vi "niFpgaDiscreteControlFilterTemplate.vi"(0 "input":fxp<+/-,16,16>, 1 "reset":bool) -> (4 "output":fxp<+/-,16,16>)   [LabVIEW 2017]
doc: "Applies a fifth-order low-pass integer FIR filter to the input data. The filter cut-off frequency is 1/10 of the sample frequency of the <B>input</B>. Use the Discrete Control Filter VI to filter measured values, such as the process variable, in control applications. The data type you wire to <B>input</B> determines the <B>output</B> data type."
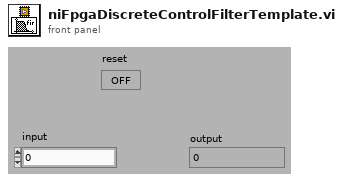
[diagram p1: front panel]
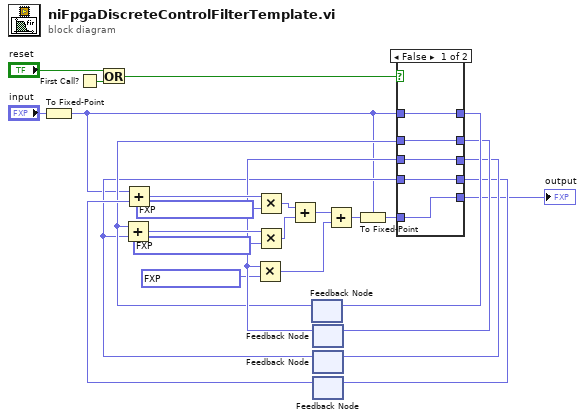
[diagram p0: block diagram]
diagram:
  n1 = To Fixed-Point(number="input") -> (fixed-point=w4:fxp<+/-,16,16>)  [unwired: 1 in]
  n2 = First Call?() -> (First Call?: T/F=w15:bool)
  n3 = Or(x="reset", y=w15) -> (x .or. y?=w16:bool)
  n4 = feedback #1() -> (w13:fxp<+/-,16,16>)  [unwired: 1 in]
  n5 = feedback #2() -> (w17:fxp<+/-,16,16>)  [unwired: 1 in]
  n6 = Multiply(x=w17, y=fxp<+,11,-2> 0.2398681640625) -> (x*y=w7:fxp<+/-,27,14>)
  n7 = feedback #3() -> (w12:fxp<+/-,16,16>)  [unwired: 1 in]
  n8 = Add(x=w13, y=w12) -> (x+y=w19:fxp<+/-,17,17>)
  n9 = Multiply(x=w19, y=fxp<+,14,-2> 0.2356414794921875) -> (x*y=w18:fxp<+/-,31,15>)
  n10 = feedback #4() -> (w14:fxp<+/-,16,16>)  [unwired: 1 in]
  n11 = Add(x=w4, y=w14) -> (x+y=w21:fxp<+/-,17,17>)
  n12 = Multiply(x=w21, y=fxp<+,14,-2> 0.1444244384765625) -> (x*y=w20:fxp<+/-,31,15>)
  n13 = Add(x=w20, y=w18) -> (x+y=w8:fxp<+/-,32,16>)
  n14 = Add(x=w8, y=w7) -> (x+y=w6:fxp<+/-,32,16>)
  n15 = To Fixed-Point(fixed-point type=w4, number=w6) -> (fixed-point=w11:fxp<+/-,16,16>)
  n16 = case shown="False" w16 {
    tunnel: [w30 w31] -> w25
    tunnel: w4 -> [w30 w31]
    tunnel: [w29 w31] -> w24
    tunnel: [w28 w31] -> w23
    tunnel: [w27 w31] -> w22
    tunnel: w17 -> [w28 _]
    tunnel: w12 -> [w27 _]
    tunnel: w13 -> [w29 _]
    tunnel: w11 -> [w26 _]
    tunnel: [w26 w31] -> w9
    frame False {
    }
    frame True {
    }
  }
  "output" <- w9
  n17 = feedback-in #1(w25) -> ()
  n18 = feedback-in #2(w24) -> ()
  n19 = feedback-in #3(w23) -> ()
  n20 = feedback-in #4(w22) -> ()
